vi "CAPA_COLOR.vi"(2 "Enum":T1(ring), 3 "24-bit pixmap":u32[][](array[numeric])) -> (0 "Array":u8[][](array[numeric]), 1 "new picture":picture)   [LabVIEW 2020]
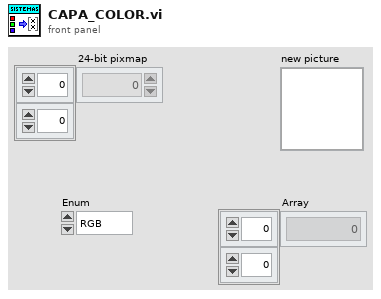
[diagram p1: front panel]
types:
  T1 = enum16{"RGB", "R", "G", "B", "C", "M", "Y", "H", "S", "V", "I", "YI", "II", "Q", ""}
  T2 = typedef "imagedata.ctl" = cluster{"image type":i32, "image depth":i32, "image":u8[], "mask":u8[], "colors":u32[], "Rectangle":cluster{"left":i16, "top":i16, "right":i16, "bottom":i16}}
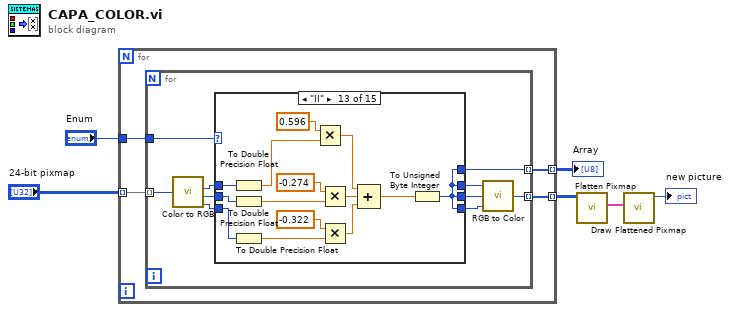
[diagram p0: block diagram]
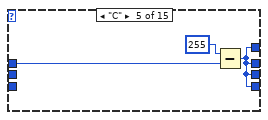
[diagram p6: hidden frame]
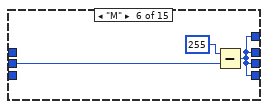
[diagram p7: hidden frame]
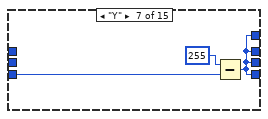
[diagram p8: hidden frame]
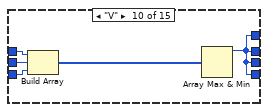
[diagram p11: hidden frame]
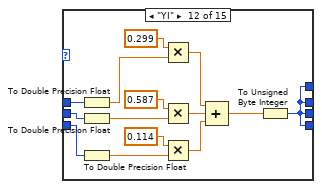
[diagram p13: hidden frame]
diagram:
  n1 = for {
    tunnel: [w10] -> w3 mode=indexing
    tunnel: "24-bit pixmap" -> [w9] mode=indexing
    tunnel: "Enum" -> [w8]
    tunnel: [w7] -> w6 mode=indexing
    n2 = for {
      tunnel: [w20] -> w10 mode=indexing
      tunnel: w9 -> [w19] mode=indexing
      tunnel: w8 -> [w18]
      tunnel: [w11] -> w7 mode=indexing
      n3 = call <vilib>:"Color to RGB.vi"("Color"=w19) -> ("R"=w16:u8, "G"=w14:u8, "B"=w13:u8)  [unwired: 1 out]
      n4 = case shown="\"II\"" w18 {
        tunnel: [w23 w24 w25 w26 w27 w30 w33 _ _ w36 _ w41 w58 _ _] -> w17
        tunnel: w16 -> [w23 w24 _ _ w29 _ _ _ _ w40 _ w54 w57 _ _]
        tunnel: [w22 w24 w25 w26 w27 w30 w33 _ _ w36 _ w41 w58 _ _] -> w15
        tunnel: w14 -> [w22 _ w25 _ _ w31 _ _ _ w39 _ w52 w56 _ _]
        tunnel: w13 -> [w21 _ _ w26 _ _ w34 _ _ w38 _ w53 w55 _ _]
        tunnel: [w21 w24 w25 w26 w27 w30 w33 _ _ w36 _ w41 w58 _ _] -> w12
        tunnel: [_ w24 w25 w26 w27 w30 w33 _ _ w36 _ w41 w58 _ _] -> w11
        frame "RGB", Default {
        }
        frame "R" {
        }
        frame "G" {
        }
        frame "B" {
        }
        frame "C" {
          n5 = Subtract(x=u8 255, y=w29) -> (x-y=w27:u8)
        }
        frame "M" {
          n6 = Subtract(x=u8 255, y=w31) -> (x-y=w30:u8)
        }
        frame "Y" {
          n7 = Subtract(x=u8 255, y=w34) -> (x-y=w33:u8)
        }
        frame "H" {
        }
        frame "S" {
        }
        frame "V" {
          n8 = Build Array(w40, w39, w38) -> (w37:u8[])
          n9 = Array Max & Min(array=w37) -> (max value=w36:u8)  [unwired: 3 out]
        }
        frame "I" {
        }
        frame "YI" {
          n10 = To Double Precision Float(number=w54) -> (double precision float=w51:dbl)
          n11 = To Double Precision Float(number=w52) -> (double precision float=w50:dbl)
          n12 = To Double Precision Float(number=w53) -> (double precision float=w49:dbl)
          n13 = Multiply(x=0.299, y=w51) -> (x*y=w45:dbl)
          n14 = Multiply(x=0.587, y=w50) -> (x*y=w44:dbl)
          n15 = Multiply(x=0.114, y=w49) -> (x*y=w43:dbl)
          n16 = Compound Arithmetic op=ADD(w45, w44, w43) -> (w42:dbl)
          n17 = To Unsigned Byte Integer(number=w42) -> (unsigned 8bit integer=w41:u8)
        }
        frame "II" {
          n18 = To Double Precision Float(number=w57) -> (double precision float=w62:dbl)
          n19 = To Double Precision Float(number=w56) -> (double precision float=w63:dbl)
          n20 = To Double Precision Float(number=w55) -> (double precision float=w64:dbl)
          n21 = Multiply(x=0.596, y=w62) -> (x*y=w65:dbl)
          n22 = Multiply(x=-0.274, y=w63) -> (x*y=w66:dbl)
          n23 = Multiply(x=-0.322, y=w64) -> (x*y=w67:dbl)
          n24 = Compound Arithmetic op=ADD(w65, w66, w67) -> (w68:dbl)
          n25 = To Unsigned Byte Integer(number=w68) -> (unsigned 8bit integer=w58:u8)
        }
        frame "Q" {
        }
        frame "" {
        }
      }
      n26 = call <vilib>:"RGB to Color.vi"("B"=w12, "G"=w15, "R"=w17) -> ("Color"=w20:u32)
    }
  }
  "Array" <- w6
  n27 = call <vilib>:"Flatten Pixmap.vi"("24-bit pixmap"=w3) -> ("image data"=w1:T2)  [unwired: 10 in]
  n28 = call <vilib>:"Draw Flattened Pixmap.vi"("image data"=w1) -> ("new picture"=→"new picture":picture)  [unwired: 8 in]
